vi "setConfigArrayT.vi"(8 "error in (no error)":errorcluster, 10 "ConfigArray":T1(array[cluster]), 11 "K2602 in":refnum<class "K2602.lvclass">) -> (0 "error out":errorcluster, 3 "K2602 out":refnum<class "K2602.lvclass">)   [LabVIEW 2009, in "Hardware.lvlib" / "Channels.lvlib" / "K2602.lvclass"]
uses:
  K2602.lvclass
  K2602.lvclass/K2602.ctl
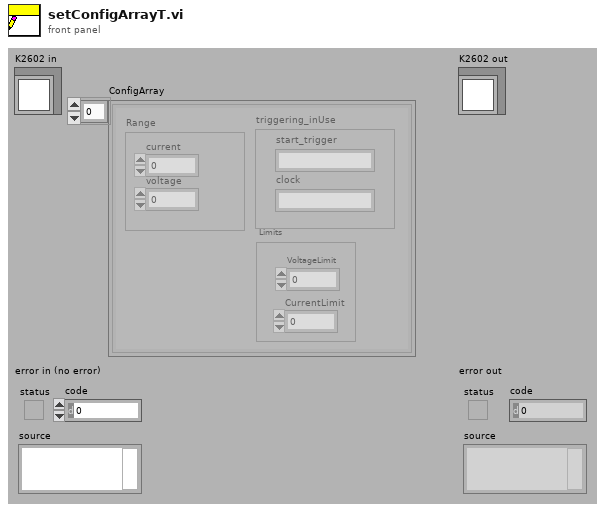
[diagram p1: front panel]
types:
  T1 = cluster{"Range":cluster{"current":dbl, "voltage":dbl}, "triggering_inUse":cluster{"start_trigger":string, "clock":string}, "Limits":cluster{"VoltageLimit":dbl, "CurrentLimit":dbl}}[]
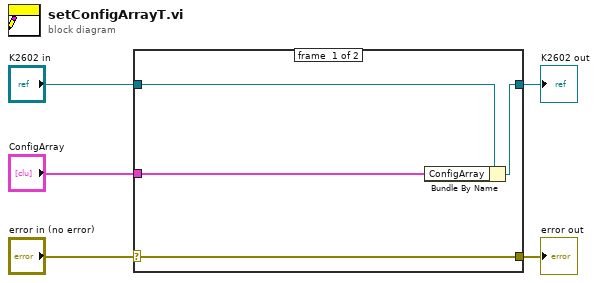
[diagram p0: block diagram]
diagram:
  n1 = case shown="No Error" "error in (no error)" {
    selector: "error in (no error)" -> [w9 w10]
    tunnel: [w9 w10] -> w4
    tunnel: [w7 w11] -> w2
    tunnel: "K2602 in" -> [w8 w11]
    tunnel: "ConfigArray" -> [w6 _]
    frame #0 {
      n2 = Bundle By Name(cluster=w8, "ConfigArray"=w6) -> (w7:refnum<class "K2602.lvclass">)
    }
    frame #1 {
    }
  }
  "error out" <- w4
  "K2602 out" <- w2
